vi "FipsAdjacent.vi"() -> (11 "Fips":i32[](array[numeric]))   [LabVIEW 2017] (continued)
 County, TX\"\t48317\n\"Glasscock County, TX\"\t48173\t\"Midland County, TX\"\t48329\n\"Glasscock County, TX\"\t48173\t\"Reagan County, TX\"\t48383\n\"Glasscock County, TX\"\t48173\t\"Sterling County, TX\"\t48431\n\"Glasscock County, TX\"\t48173\t\"Upton County, TX\"\t48461\n\"Goliad County, TX\"\t48175\t\"Bee County, TX\"\t48025\n\"Goliad County, TX\"\t48175\t\"DeWitt County, TX\"\t48123\n\"Goliad County, TX\"\t48175\t\"Goliad County, TX\"\t48175\n\"Goliad County, TX\"\t48175\t\"Karnes County, TX\"\t48255\n\"Goliad County, TX\"\t48175\t\"Refugio County, TX\"\t48391\n\"Goliad County, TX\"\t48175\t\"Victoria County, TX\"\t48469\n\"Gonzales County, TX\"\t48177\t\"Caldwell County, TX\"\t48055\n\"Gonzales County, TX\"\t48177\t\"DeWitt County, TX\"\t48123\n\"Gonzales County, TX\"\t48177\t\"Fayette County, TX\"\t48149\n\"Gonzales County, TX\"\t48177\t\"Gonzales County, TX\"\t48177\n\"Gonzales County, TX\"\t48177\t\"Guadalupe County, TX\"\t48187\n\"Gonzales County, TX\"\t48177\t\"Karnes County, TX\"\t48255\n\"Gonzales County, TX\"\t48177\t\"Lavaca County, TX\"\t48285\n\"Gonzales County, TX\"\t48177\t\"Wilson County, TX\"\t48493\n\"Gray County, TX\"\t48179\t\"Armstrong County, TX\"\t48011\n\"Gray County, TX\"\t48179\t\"Carson County, TX\"\t48065\n\"Gray County, TX\"\t48179\t\"Collingsworth County, TX\"\t48087\n\"Gray County, TX\"\t48179\t\"Donley County, TX\"\t48129\n\"Gray County, TX\"\t48179\t\"Gray County, TX\"\t48179\n\"Gray County, TX\"\t48179\t\"Hemphill County, TX\"\t48211\n\"Gray County, TX\"\t48179\t\"Roberts County, TX\"\t48393\n\"Gray County, TX\"\t48179\t\"Wheeler County, TX\"\t48483\n\"Grayson County, TX\"\t48181\t\"Bryan County, OK\"\t40013\n\"Grayson County, TX\"\t48181\t\"Love County, OK\"\t40085\n\"Grayson County, TX\"\t48181\t\"Marshall County, OK\"\t40095\n\"Grayson County, TX\"\t48181\t\"Collin County, TX\"\t48085\n\"Grayson County, TX\"\t48181\t\"Cooke County, TX\"\t48097\n\"Grayson County, TX\"\t48181\t\"Denton County, TX\"\t48121\n\"Grayson County, TX\"\t48181\t\"Fannin County, TX\"\t48147\n\"Grayson County, TX\"\t48181\t\"Grayson County, TX\"\t48181\n\"Gregg County, TX\"\t48183\t\"Gregg County, TX\"\t48183\n\"Gregg County, TX\"\t48183\t\"Harrison County, TX\"\t48203\n\"Gregg County, TX\"\t48183\t\"Rusk County, TX\"\t48401\n\"Gregg County, TX\"\t48183\t\"Smith County, TX\"\t48423\n\"Gregg County, TX\"\t48183\t\"Upshur County, TX\"\t48459\n\"Grimes County, TX\"\t48185\t\"Brazos County, TX\"\t48041\n\"Grimes County, TX\"\t48185\t\"Grimes County, TX\"\t48185\n\"Grimes County, TX\"\t48185\t\"Madison County, TX\"\t48313\n\"Grimes County, TX\"\t48185\t\"Montgomery County, TX\"\t48339\n\"Grimes County, TX\"\t48185\t\"Walker County, TX\"\t48471\n\"Grimes County, TX\"\t48185\t\"Waller County, TX\"\t48473\n\"Grimes County, TX\"\t48185\t\"Washington County, TX\"\t48477\n\"Guadalupe County, TX\"\t48187\t\"Bexar County, TX\"\t48029\n\"Guadalupe County, TX\"\t48187\t\"Caldwell County, TX\"\t48055\n\"Guadalupe County, TX\"\t48187\t\"Comal County, TX\"\t48091\n\"Guadalupe County, TX\"\t48187\t\"Gonzales County, TX\"\t48177\n\"Guadalupe County, TX\"\t48187\t\"Guadalupe County, TX\"\t48187\n\"Guadalupe County, TX\"\t48187\t\"Hays County, TX\"\t48209\n\"Guadalupe County, TX\"\t48187\t\"Wilson County, TX\"\t48493\n\"Hale County, TX\"\t48189\t\"Castro County, TX\"\t48069\n\"Hale County, TX\"\t48189\t\"Crosby County, TX\"\t48107\n\"Hale County, TX\"\t48189\t\"Floyd County, TX\"\t48153\n\"Hale County, TX\"\t48189\t\"Hale County, TX\"\t48189\n\"Hale County, TX\"\t48189\t\"Hockley County, TX\"\t48219\n\"Hale County, TX\"\t48189\t\"Lamb County, TX\"\t48279\n\"Hale County, TX\"\t48189\t\"Lubbock County, TX\"\t48303\n\"Hale County, TX\"\t48189\t\"Swisher County, TX\"\t48437\n\"Hall County, TX\"\t48191\t\"Briscoe County, TX\"\t48045\n\"Hall County, TX\"\t48191\t\"Childress County, TX\"\t48075\n\"Hall County, TX\"\t48191\t\"Collingsworth County, TX\"\t48087\n\"Hall County, TX\"\t48191\t\"Cottle County, TX\"\t48101\n\"Hall County, TX\"\t48191\t\"Donley County, TX\"\t48129\n\"Hall County, TX\"\t48191\t\"Hall County, TX\"\t48191\n\"Hall County, TX\"\t48191\t\"Motley County, TX\"\t48345\n\"Hamilton County, TX\"\t48193\t\"Bosque County, TX\"\t48035\n\"Hamilton County, TX\"\t48193\t\"Comanche County, TX\"\t48093\n\"Hamilton County, TX\"\t48193\t\"Coryell County, TX\"\t48099\n\"Hamilton County, TX\"\t48193\t\"Erath County, TX\"\t48143\n\"Hamilton County, TX\"\t48193\t\"Hamilton County, TX\"\t48193\n\"Hamilton County, TX\"\t48193\t\"Lampasas County, TX\"\t48281\n\"Hamilton County, TX\"\t48193\t\"Mills County, TX\"\t48333\n\"Hansford County, TX\"\t48195\t\"Texas County, OK\"\t40139\n\"Hansford County, TX\"\t48195\t\"Hansford County, TX\"\t48195\n\"Hansford County, TX\"\t48195\t\"Hutchinson County, TX\"\t48233\n\"Hansford County, TX\"\t48195\t\"Moore County, TX\"\t48341\n\"Hansford County, TX\"\t48195\t\"Ochiltree County, TX\"\t48357\n\"Hansford County, TX\"\t48195\t\"Roberts County, TX\"\t48393\n\"Hansford County, TX\"\t48195\t\"Sherman County, TX\"\t48421\n\"Hardeman County, TX\"\t48197\t\"Harmon County, OK\"\t40057\n\"Hardeman County, TX\"\t48197\t\"Jackson County, OK\"\t40065\n\"Hardeman County, TX\"\t48197\t\"Childress County, TX\"\t48075\n\"Hardeman County, TX\"\t48197\t\"Cottle County, TX\"\t48101\n\"Hardeman County, TX\"\t48197\t\"Foard County, TX\"\t48155\n\"Hardeman County, TX\"\t48197\t\"Hardeman County, TX\"\t48197\n\"Hardeman County, TX\"\t48197\t\"Wilbarger County, TX\"\t48487\n\"Hardin County, TX\"\t48199\t\"Hardin County, TX\"\t48199\n\"Hardin County, TX\"\t48199\t\"Jasper County, TX\"\t48241\n\"Hardin County, TX\"\t48199\t\"Jefferson County, TX\"\t48245\n\"Hardin County, TX\"\t48199\t\"Liberty County, TX\"\t48291\n\"Hardin County, TX\"\t48199\t\"Orange County, TX\"\t48361\n\"Hardin County, TX\"\t48199\t\"Polk County, TX\"\t48373\n\"Hardin County, TX\"\t48199\t\"Tyler County, TX\"\t48457\n\"Harris County, TX\"\t48201\t\"Brazoria County, TX\"\t48039\n\"Harris County, TX\"\t48201\t\"Chambers County, TX\"\t48071\n\"Harris County, TX\"\t48201\t\"Fort Bend County, TX\"\t48157\n\"Harris County, TX\"\t48201\t\"Galveston County, TX\"\t48167\n\"Harris County, TX\"\t48201\t\"Harris County, TX\"\t48201\n\"Harris County, TX\"\t48201\t\"Liberty County, TX\"\t48291\n\"Harris County, TX\"\t48201\t\"Montgomery County, TX\"\t48339\n\"Harris County, TX\"\t48201\t\"Waller County, TX\"\t48473\n\"Harrison County, TX\"\t48203\t\"Caddo Parish, LA\"\t22017\n\"Harrison County, TX\"\t48203\t\"Gregg County, TX\"\t48183\n\"Harrison County, TX\"\t48203\t\"Harrison County, TX\"\t48203\n\"Harrison County, TX\"\t48203\t\"Marion County, TX\"\t48315\n\"Harrison County, TX\"\t48203\t\"Panola County, TX\"\t48365\n\"Harrison County, TX\"\t48203\t\"Rusk County, TX\"\t48401\n\"Harrison County, TX\"\t48203\t\"Upshur County, TX\"\t48459\n\"Hartley County, TX\"\t48205\t\"Quay County, NM\"\t35037\n\"Hartley County, TX\"\t48205\t\"Union County, NM\"\t35059\n\"Hartley County, TX\"\t48205\t\"Dallam County, TX\"\t48111\n\"Hartley County, TX\"\t48205\t\"Hartley County, TX\"\t48205\n\"Hartley County, TX\"\t48205\t\"Moore County, TX\"\t48341\n\"Hartley County, TX\"\t48205\t\"Oldham County, TX\"\t48359\n\"Hartley County, TX\"\t48205\t\"Sherman County, TX\"\t48421\n\"Haskell County, TX\"\t48207\t\"Baylor County, TX\"\t48023\n\"Haskell County, TX\"\t48207\t\"Haskell County, TX\"\t48207\n\"Haskell County, TX\"\t48207\t\"Jones County, TX\"\t48253\n\"Haskell County, TX\"\t48207\t\"King County, TX\"\t48269\n\"Haskell County, TX\"\t48207\t\"Knox County, TX\"\t48275\n\"Haskell County, TX\"\t48207\t\"Shackelford County, TX\"\t48417\n\"Haskell County, TX\"\t48207\t\"Stonewall County, TX\"\t48433\n\"Haskell County, TX\"\t48207\t\"Throckmorton County, TX\"\t48447\n\"Hays County, TX\"\t48209\t\"Blanco County, TX\"\t48031\n\"Hays County, TX\"\t48209\t\"Caldwell County, TX\"\t48055\n\"Hays County, TX\"\t48209\t\"Comal County, TX\"\t48091\n\"Hays County, TX\"\t48209\t\"Guadalupe County, TX\"\t48187\n\"Hays County, TX\"\t48209\t\"Hays County, TX\"\t48209\n\"Hays County, TX\"\t48209\t\"Travis County, TX\"\t48453\n\"Hemphill County, TX\"\t48211\t\"Ellis County, OK\"\t40045\n\"Hemphill County, TX\"\t48211\t\"Roger Mills County, OK\"\t40129\n\"Hemphill County, TX\"\t48211\t\"Gray County, TX\"\t48179\n\"Hemphill County, TX\"\t48211\t\"Hemphill County, TX\"\t48211\n\"Hemphill County, TX\"\t48211\t\"Lipscomb County, TX\"\t48295\n\"Hemphill County, TX\"\t48211\t\"Roberts County, TX\"\t48393\n\"Hemphill County, TX\"\t48211\t\"Wheeler County, TX\"\t48483\n\"Henderson County, TX\"\t48213\t\"Anderson County, TX\"\t48001\n\"Henderson County, TX\"\t48213\t\"Cherokee County, TX\"\t48073\n\"Henderson County, TX\"\t48213\t\"Ellis County, TX\"\t48139\n\"Henderson County, TX\"\t48213\t\"Freestone County, TX\"\t48161\n\"Henderson County, TX\"\t48213\t\"Henderson County, TX\"\t48213\n\"Henderson County, TX\"\t48213\t\"Kaufman County, TX\"\t48257\n\"Henderson County, TX\"\t48213\t\"Navarro County, TX\"\t48349\n\"Henderson County, TX\"\t48213\t\"Smith County, TX\"\t48423\n\"Henderson County, TX\"\t48213\t\"Van Zandt County, TX\"\t48467\n\"Hidalgo County, TX\"\t48215\t\"Brooks County, TX\"\t48047\n\"Hidalgo County, TX\"\t48215\t\"Cameron County, TX\"\t48061\n\"Hidalgo County, TX\"\t48215\t\"Hidalgo County, TX\"\t48215\n\"Hidalgo County, TX\"\t48215\t\"Kenedy County, TX\"\t48261\n\"Hidalgo County, TX\"\t48215\t\"Starr County, TX\"\t48427\n\"Hidalgo County, TX\"\t48215\t\"Willacy County, TX\"\t48489\n\"Hill County, TX\"\t48217\t\"Bosque County, TX\"\t48035\n\"Hill County, TX\"\t48217\t\"Ellis County, TX\"\t48139\n\"Hill County, TX\"\t48217\t\"Hill County, TX\"\t48217\n\"Hill County, TX\"\t48217\t\"Johnson County, TX\"\t48251\n\"Hill County, TX\"\t48217\t\"Limestone County, TX\"\t48293\n\"Hill County, TX\"\t48217\t\"McLennan County, TX\"\t48309\n\"Hill County, TX\"\t48217\t\"Navarro County, TX\"\t48349\n\"Hockley County, TX\"\t48219\t\"Bailey County, TX\"\t48017\n\"Hockley County, TX\"\t48219\t\"Cochran County, TX\"\t48079\n\"Hockley County, TX\"\t48219\t\"Hale County, TX\"\t48189\n\"Hockley County, TX\"\t48219\t\"Hockley County, TX\"\t48219\n\"Hockley County, TX\"\t48219\t\"Lamb County, TX\"\t48279\n\"Hockley County, TX\"\t48219\t\"Lubbock County, TX\"\t48303\n\"Hockley County, TX\"\t48219\t\"Lynn County, TX\"\t48305\n\"Hockley County, TX\"\t48219\t\"Terry County, TX\"\t48445\n\"Hockley County, TX\"\t48219\t\"Yoakum County, TX\"\t48501\n\"Hood County, TX\"\t48221\t\"Erath County, TX\"\t48143\n\"Hood County, TX\"\t48221\t\"Hood County, TX\"\t48221\n\"Hood County, TX\"\t48221\t\"Johnson County, TX\"\t48251\n\"Hood County, TX\"\t48221\t\"Palo Pinto County, TX\"\t48363\n\"Hood County, TX\"\t48221\t\"Parker County, TX\"\t48367\n\"Hood County, TX\"\t48221\t\"Somervell County, TX\"\t48425\n\"Hopkins County, TX\"\t48223\t\"Delta County, TX\"\t48119\n\"Hopkins County, TX\"\t48223\t\"Franklin County, TX\"\t48159\n\"Hopkins County, TX\"\t48223\t\"Hopkins County, TX\"\t48223\n\"Hopkins County, TX\"\t48223\t\"Hunt County, TX\"\t48231\n\"Hopkins County, TX\"\t48223\t\"Rains County, TX\"\t48379\n\"Hopkins County, TX\"\t48223\t\"Wood County, TX\"\t48499\n\"Houston County, TX\"\t48225\t\"Anderson County, TX\"\t48001\n\"Houston County, TX\"\t48225\t\"Angelina County, TX\"\t48005\n\"Houston County, TX\"\t48225\t\"Cherokee County, TX\"\t48073\n\"Houston County, TX\"\t48225\t\"Houston County, TX\"\t48225\n\"Houston County, TX\"\t48225\t\"Leon County, TX\"\t48289\n\"Houston County, TX\"\t48225\t\"Madison County, TX\"\t48313\n\"Houston County, TX\"\t48225\t\"Trinity County, TX\"\t48455\n\"Houston County, TX\"\t48225\t\"Walker County, TX\"\t48471\n\"Howard County, TX\"\t48227\t\"Borden County, TX\"\t48033\n\"Howard County, TX\"\t48227\t\"Dawson County, TX\"\t48115\n\"Howard County, TX\"\t48227\t\"Glasscock County, TX\"\t48173\n\"Howard County, TX\"\t48227\t\"Howard County, TX\"\t48227\n\"Howard County, TX\"\t48227\t\"Martin County, TX\"\t48317\n\"Howard County, TX\"\t48227\t\"Mitchell County, TX\"\t48335\n\"Howard County, TX\"\t48227\t\"Sterling County, TX\"\t48431\n\"Hudspeth County, TX\"\t48229\t\"Otero County, NM\"\t35035\n\"Hudspeth County, TX\"\t48229\t\"Culberson County, TX\"\t48109\n\"Hudspeth County, TX\"\t48229\t\"El Paso County, TX\"\t48141\n\"Hudspeth County, TX\"\t48229\t\"Hudspeth County, TX\"\t48229\n\"Hudspeth County, TX\"\t48229\t\"Jeff Davis County, TX\"\t48243\n\"Hudspeth County, TX\"\t48229\t\"Presidio County, TX\"\t48377\n\"Hunt County, TX\"\t48231\t\"Collin County, TX\"\t48085\n\"Hunt County, TX\"\t48231\t\"Delta County, TX\"\t48119\n\"Hunt County, TX\"\t48231\t\"Fannin County, TX\"\t48147\n\"Hunt County, TX\"\t48231\t\"Hopkins County, TX\"\t48223\n\"Hunt County, TX\"\t48231\t\"Hunt County, TX\"\t48231\n\"Hunt County, TX\"\t48231\t\"Kaufman County, TX\"\t48257\n\"Hunt County, TX\"\t48231\t\"Rains County, TX\"\t48379\n\"Hunt County, TX\"\t48231\t\"Rockwall County, TX\"\t48397\n\"Hunt County, TX\"\t48231\t\"Van Zandt County, TX\"\t48467\n\"Hutchinson County, TX\"\t48233\t\"Carson County, TX\"\t48065\n\"Hutchinson County, TX\"\t48233\t\"Hansford County, TX\"\t48195\n\"Hutchinson County, TX\"\t48233\t\"Hutchinson County, TX\"\t48233\n\"Hutchinson County, TX\"\t48233\t\"Moore County, TX\"\t48341\n\"Hutchinson County, TX\"\t48233\t\"Roberts County, TX\"\t48393\n\"Hutchinson County, TX\"\t48233\t\"Sherman County, TX\"\t48421\n\"Irion County, TX\"\t48235\t\"Crockett County, TX\"\t48105\n\"Irion County, TX\"\t48235\t\"Irion County, TX\"\t48235\n\"Irion County, TX\"\t48235\t\"Reagan County, TX\"\t48383\n\"Irion County, TX\"\t48235\t\"Schleicher County, TX\"\t48413\n\"Irion County, TX\"\t48235\t\"Tom Green County, TX\"\t48451\n\"Jack County, TX\"\t48237\t\"Archer County, TX\"\t48009\n\"Jack County, TX\"\t48237\t\"Clay County, TX\"\t48077\n\"Jack County, TX\"\t48237\t\"Jack County, TX\"\t48237\n\"Jack County, TX\"\t48237\t\"Montague County, TX\"\t48337\n\"Jack County, TX\"\t48237\t\"Palo Pinto County, TX\"\t48363\n\"Jack County, TX\"\t48237\t\"Parker County, TX\"\t48367\n\"Jack County, TX\"\t48237\t\"Wise County, TX\"\t48497\n\"Jack County, TX\"\t48237\t\"Young County, TX\"\t48503\n\"Jackson County, TX\"\t48239\t\"Calhoun County, TX\"\t48057\n\"Jackson County, TX\"\t48239\t\"Colorado County, TX\"\t48089\n\"Jackson County, TX\"\t48239\t\"Jackson County, TX\"\t48239\n\"Jackson County, TX\"\t48239\t\"Lavaca County, TX\"\t48285\n\"Jackson County, TX\"\t48239\t\"Matagorda County, TX\"\t48321\n\"Jackson County, TX\"\t48239\t\"Victoria County, TX\"\t48469\n\"Jackson County, TX\"\t48239\t\"Wharton County, TX\"\t48481\n\"Jasper County, TX\"\t48241\t\"Angelina County, TX\"\t48005\n\"Jasper County, TX\"\t48241\t\"Hardin County, TX\"\t48199\n\"Jasper County, TX\"\t48241\t\"Jasper County, TX\"\t48241\n\"Jasper County, TX\"\t48241\t\"Newton County, TX\"\t48351\n\"Jasper County, TX\"\t48241\t\"Orange County, TX\"\t48361\n\"Jasper County, TX\"\t48241\t\"Sabine County, TX\"\t48403\n\"Jasper County, TX\"\t48241\t\"San Augustine County, TX\"\t48405\n\"Jasper County, TX\"\t48241\t\"Tyler County, TX\"\t48457\n\"Jeff Davis County, TX\"\t48243\t\"Brewster County, TX\"\t48043\n\"Jeff Davis County, TX\"\t48243\t\"Culberson County, TX\"\t48109\n\"Jeff Davis County, TX\"\t48243\t\"Hudspeth County, TX\"\t48229\n\"Jeff Davis County, TX\"\t48243\t\"Jeff Davis County, TX\"\t48243\n\"Jeff Davis County, TX\"\t48243\t\"Pecos County, TX\"\t48371\n\"Jeff Davis County, TX\"\t48243\t\"Presidio County, TX\"\t48377\n\"Jeff Davis County, TX\"\t48243\t\"Reeves County, TX\"\t48389\n\"Jefferson County, TX\"\t48245\t\"Cameron Parish, LA\"\t22023\n\"Jefferson County, TX\"\t48245\t\"Chambers County, TX\"\t48071\n\"Jefferson County, TX\"\t48245\t\"Hardin County, TX\"\t48199\n\"Jefferson County, TX\"\t48245\t\"Jefferson County, TX\"\t48245\n\"Jefferson County, TX\"\t48245\t\"Liberty County, TX\"\t48291\n\"Jefferson County, TX\"\t48245\t\"Orange County, TX\"\t48361\n\"Jim Hogg County, TX\"\t48247\t\"Brooks County, TX\"\t48047\n\"Jim Hogg County, TX\"\t48247\t\"Duval County, TX\"\t48131\n\"Jim Hogg County, TX\"\t48247\t\"Jim Hogg County, TX\"\t48247\n\"Jim Hogg County, TX\"\t48247\t\"Starr County, TX\"\t48427\n\"Jim Hogg County, TX\"\t48247\t\"Webb County, TX\"\t48479\n\"Jim Hogg County, TX\"\t48247\t\"Zapata County, TX\"\t48505\n\"Jim Wells County, TX\"\t48249\t\"Brooks County, TX\"\t48047\n\"Jim Wells County, TX\"\t48249\t\"Duval County, TX\"\t48131\n\"Jim Wells County, TX\"\t48249\t\"Jim Wells County, TX\"\t48249\n\"Jim Wells County, TX\"\t48249\t\"Kleberg County, TX\"\t48273\n\"Jim Wells County, TX\"\t48249\t\"Live Oak County, TX\"\t48297\n\"Jim Wells County, TX\"\t48249\t\"Nueces County, TX\"\t48355\n\"Jim Wells County, TX\"\t48249\t\"San Patricio County, TX\"\t48409\n\"Johnson County, TX\"\t48251\t\"Bosque County, TX\"\t48035\n\"Johnson County, TX\"\t48251\t\"Ellis County, TX\"\t48139\n\"Johnson County, TX\"\t48251\t\"Hill County, TX\"\t48217\n\"Johnson County, TX\"\t48251\t\"Hood County, TX\"\t48221\n\"Johnson County, TX\"\t48251\t\"Johnson County, TX\"\t48251\n\"Johnson County, TX\"\t48251\t\"Parker County, TX\"\t48367\n\"Johnson County, TX\"\t48251\t\"Somervell County, TX\"\t48425\n\"Johnson County, TX\"\t48251\t\"Tarrant County, TX\"\t48439\n\"Jones County, TX\"\t48253\t\"Callahan County, TX\"\t48059\n\"Jones County, TX\"\t48253\t\"Fisher County, TX\"\t48151\n\"Jones County, TX\"\t48253\t\"Haskell County, TX\"\t48207\n\"Jones County, TX\"\t48253\t\"Jones County, TX\"\t48253\n\"Jones County, TX\"\t48253\t\"Nolan County, TX\"\t48353\n\"Jones County, TX\"\t48253\t\"Shackelford County, TX\"\t48417\n\"Jones County, TX\"\t48253\t\"Stonewall County, TX\"\t48433\n\"Jones County, TX\"\t48253\t\"Taylor County, TX\"\t48441\n\"Karnes County, TX\"\t48255\t\"Atascosa County, TX\"\t48013\n\"Karnes County, TX\"\t48255\t\"Bee County, TX\"\t48025\n\"Karnes County, TX\"\t48255\t\"DeWitt County, TX\"\t48123\n\"Karnes County, TX\"\t48255\t\"Goliad County, TX\"\t48175\n\"Karnes County, TX\"\t48255\t\"Gonzales County, TX\"\t48177\n\"Karnes County, TX\"\t48255\t\"Karnes County, TX\"\t48255\n\"Karnes County, TX\"\t48255\t\"Live Oak County, TX\"\t48297\n\"Karnes County, TX\"\t48255\t\"Wilson County, TX\"\t48493\n\"Kaufman County, TX\"\t48257\t\"Dallas County, TX\"\t48113\n\"Kaufman County, TX\"\t48257\t\"Ellis County, TX\"\t48139\n\"Kaufman County, TX\"\t48257\t\"Henderson County, TX\"\t48213\n\"Kaufman County, TX\"\t48257\t\"Hunt County, TX\"\t48231\n\"Kaufman County, TX\"\t48257\t\"Kaufman County, TX\"\t48257\n\"Kaufman County, TX\"\t48257\t\"Rockwall County, TX\"\t48397\n\"Kaufman County, TX\"\t48257\t\"Van Zandt County, TX\"\t48467\n\"Kendall County, TX\"\t48259\t\"Bandera County, TX\"\t48019\n\"Kendall County, TX\"\t48259\t\"Bexar County, TX\"\t48029\n\"Kendall County, TX\"\t48259\t\"Blanco County, TX\"\t48031\n\"Kendall County, TX\"\t48259\t\"Comal County, TX\"\t48091\n\"Kendall County, TX\"\t48259\t\"Gillespie County, TX\"\t48171\n\"Kendall County, TX\"\t48259\t\"Kendall County, TX\"\t48259\n\"Kendall County, TX\"\t48259\t\"Kerr County, TX\"\t48265\n\"Kenedy County, TX\"\t48261\t\"Brooks County, TX\"\t48047\n\"Kenedy County, TX\"\t48261\t\"Hidalgo County, TX\"\t48215\n\"Kenedy County, TX\"\t48261\t\"Kenedy County, TX\"\t48261\n\"Kenedy County, TX\"\t48261\t\"Kleberg County, TX\"\t48273\n\"Kenedy County, TX\"\t48261\t\"Willacy County, TX\"\t48489\n\"Kent County, TX\"\t48263\t\"Crosby County, TX\"\t48107\n\"Kent County, TX\"\t48263\t\"Dickens County, TX\"\t48125\n\"Kent County, TX\"\t48263\t\"Fisher County, TX\"\t48151\n\"Kent County, TX\"\t48263\t\"Garza County, TX\"\t48169\n\"Kent County, TX\"\t48263\t\"Kent County, TX\"\t48263\n\"Kent County, TX\"\t48263\t\"King County, TX\"\t48269\n\"Kent County, TX\"\t48263\t\"Scurry County, TX\"\t48415\n\"Kent County, TX\"\t48263\t\"Stonewall County, TX\"\t48433\n\"Kerr County, TX\"\t48265\t\"Bandera County, TX\"\t48019\n\"Kerr County, TX\"\t48265\t\"Edwards County, TX\"\t48137\n\"Kerr County, TX\"\t48265\t\"Gillespie County, TX\"\t48171\n\"Kerr County, TX\"\t48265\t\"Kendall County, TX\"\t48259\n\"Kerr County, TX\"\t48265\t\"Kerr County, TX\"\t48265\n\"Kerr County, TX\"\t48265\t\"Kimble County, TX\"\t48267\n\"Kerr County, TX\"\t48265\t\"Real County, TX\"\t48385\n\"Kimble County, TX\"\t48267\t\"Edwards County, TX\"\t48137\n\"Kimble County, TX\"\t48267\t\"Gillespie County, TX\"\t48171\n\"Kimble County, TX\"\t48267\t\"Kerr County, TX\"\t48265\n\"Kimble County, TX\"\t48267\t\"Kimble County, TX\"\t48267\n\"Kimble County, TX\"\t48267\t\"Mason County, TX\"\t48319\n\"Kimble County, TX\"\t48267\t\"Menard County, TX\"\t48327\n\"Kimble County, TX\"\t48267\t\"Schleicher County, TX\"\t48413\n\"Kimble County, TX\"\t48267\t\"Sutton County, TX\"\t48435\n\"King County, TX\"\t48269\t\"Cottle County, TX\"\t48101\n\"King County, TX\"\t48269\t\"Dickens County, TX\"\t48125\n\"King County, TX\"\t48269\t\"Foard County, TX\"\t48155\n\"King County, TX\"\t48269\t\"Haskell County, TX\"\t48207\n\"King County, TX\"\t48269\t\"Kent County, TX\"\t48263\n\"King County, TX\"\t48269\t\"King County, TX\"\t48269\n\"King County, TX\"\t48269\t\"Knox County, TX\"\t48275\n\"King County, TX\"\t48269\t\"Motley County, TX\"\t48345\n\"King County, TX\"\t48269\t\"Stonewall County, TX\"\t48433\n\"Kinney County, TX\"\t48271\t\"Edwards County, TX\"\t48137\n\"Kinney County, TX\"\t48271\t\"Kinney County, TX\"\t48271\n\"Kinney County, TX\"\t48271\t\"Maverick County, TX\"\t48323\n\"Kinney County, TX\"\t48271\t\"Uvalde County, TX\"\t48463\n\"Kinney County, TX\"\t48271\t\"Val Verde County, TX\"\t48465\n\"Kinney County, TX\"\t48271\t\"Zavala County, TX\"\t48507\n\"Kleberg County, TX\"\t48273\t\"Brooks County, TX\"\t48047\n\"Kleberg County, TX\"\t48273\t\"Jim Wells County, TX\"\t48249\n\"Kleberg County, TX\"\t48273\t\"Kenedy County, TX\"\t48261\n\"Kleberg County, TX\"\t48273\t\"Kleberg County, TX\"\t48273\n\"Kleberg County, TX\"\t48273\t\"Nueces County, TX\"\t48355\n\"Knox County, TX\"\t48275\t\"Baylor County, TX\"\t48023\n\"Knox County, TX\"\t48275\t\"Foard County, TX\"\t48155\n\"Knox County, TX\"\t48275\t\"Haskell County, TX\"\t48207\n\"Knox County, TX\"\t48275\t\"King County, TX\"\t48269\n\"Knox County, TX\"\t48275\t\"Knox County, TX\"\t48275\n\"Knox County, TX\"\t48275\t\"Stonewall County, TX\"\t48433\n\"Knox County, TX\"\t48275\t\"Throckmorton County, TX\"\t48447\n\"Lamar County, TX\"\t48277\t\"Bryan County, OK\"\t40013\n\"Lamar County, TX\"\t48277\t\"Choctaw County, OK\"\t40023\n\"Lamar County, TX\"\t48277\t\"Delta County, TX\"\t48119\n\"Lamar County, TX\"\t48277\t\"Fannin County, TX\"\t48147\n\"Lamar County, TX\"\t48277\t\"Lamar County, TX\"\t48277\n\"Lamar County, TX\"\t48277\t\"Red River County, TX\"\t48387\n\"Lamb County, TX\"\t48279\t\"Bailey County, TX\"\t48017\n\"Lamb County, TX\"\t48279\t\"Castro County, TX\"\t48069\n\"Lamb County, TX\"\t48279\t\"Cochran County, TX\"\t48079\n\"Lamb County, TX\"\t48279\t\"Hale County, TX\"\t48189\n\"Lamb County, TX\"\t48279\t\"Hockley County, TX\"\t48219\n\"Lamb County, TX\"\t48279\t\"Lamb County, TX\"\t48279\n\"Lamb County, TX\"\t48279\t\"Lubbock County, TX\"\t48303\n\"Lamb County, TX\"\t48279\t\"Parmer County, TX\"\t48369\n\"Lampasas County, TX\"\t48281\t\"Bell County, TX\"\t48027\n\"Lampasas County, TX\"\t48281\t\"Burnet County, TX\"\t48053\n\"Lampasas County, TX\"\t48281\t\"Coryell County, TX\"\t48099\n\"Lampasas County, TX\"\t48281\t\"Hamilton County, TX\"\t48193\n\"Lampasas County, TX\"\t48281\t\"Lampasas County, TX\"\t48281\n\"Lampasas County, TX\"\t48281\t\"Mills County, TX\"\t48333\n\"Lampasas County, TX\"\t48281\t\"San Saba County, TX\"\t48411\n\"La Salle County, TX\"\t48283\t\"Atascosa County, TX\"\t48013\n\"La Salle County, TX\"\t48283\t\"Dimmit County, TX\"\t48127\n\"La Salle County, TX\"\t48283\t\"Duval County, TX\"\t48131\n\"La Salle County, TX\"\t48283\t\"Frio County, TX\"\t48163\n\"La Salle County, TX\"\t48283\t\"La Salle County, TX\"\t48283\n\"La Salle County, TX\"\t48283\t\"McMullen County, TX\"\t48311\n\"La Salle County, TX\"\t48283\t\"Webb County, TX\"\t48479\n\"Lavaca County, TX\"\t48285\t\"Colorado County, TX\"\t48089\n\"Lavaca County, TX\"\t48285\t\"DeWitt County, TX\"\t48123\n\"Lavaca County, TX\"\t48285\t\"Fayette County, TX\"\t48149\n\"Lavaca County, TX\"\t48285\t\"Gonzales County, TX\"\t48177\n\"Lavaca County, TX\"\t48285\t\"Jackson County, TX\"\t48239\n\"Lavaca County, TX\"\t48285\t\"Lavaca County, TX\"\t48285\n\"Lavaca County, TX\"\t48285\t\"Victoria County, TX\"\t48469\n\"Lee County, TX\"\t48287\t\"Bastrop County, TX\"\t48021\n\"Lee County, TX\"\t48287\t\"Burleson County, TX\"\t48051\n\"Lee County, TX\"\t48287\t\"Fayette County, TX\"\t48149\n\"Lee County, TX\"\t48287\t\"Lee County, TX\"\t48287\n\"Lee County, TX\"\t48287\t\"Milam County, TX\"\t48331\n\"Lee County, TX\"\t48287\t\"Washington County, TX\"\t48477\n\"Lee County, TX\"\t48287\t\"Williamson County, TX\"\t48491\n\"Leon County, TX\"\t48289\t\"Anderson County, TX\"\t48001\n\"Leon County, TX\"\t48289\t\"Brazos County, TX\"\t48041\n\"Leon County, TX\"\t48289\t\"Freestone County, TX\"\t48161\n\"Leon County, TX\"\t48289\t\"Houston County, TX\"\t48225\n\"Leon County, TX\"\t48289\t\"Leon County, TX\"\t48289\n\"Leon County, TX\"\t48289\t\"Limestone County, TX\"\t48293\n\"Leon County, TX\"\t48289\t\"Madison County, TX\"\t48313\n\"Leon County, TX\"\t48289\t\"Robertson County, TX\"\t48395\n\"Liberty County, TX\"\t48291\t\"Chambers County, TX\"\t48071\n\"Liberty County, TX\"\t48291\t\"Hardin County, TX\"\t48199\n\"Liberty County, TX\"\t48291\t\"Harris County, TX\"\t48201\n\"Liberty County, TX\"\t48291\t\"Jefferson County, TX\"\t48245\n\"Liberty County, TX\"\t48291\t\"Liberty County, TX\"\t48291\n\"Liberty County, TX\"\t48291\t\"Montgomery County, TX\"\t48339\n\"Liberty County, TX\"\t48291\t\"Polk County, TX\"\t48373\n\"Liberty County, TX\"\t48291\t\"San Jacinto County, TX\"\t48407\n\"Limestone County, TX\"\t48293\t\"Falls County, TX\"\t48145\n\"Limestone County, TX\"\t48293\t\"Freestone County, TX\"\t48161\n\"Limestone County, TX\"\t48293\t\"Hill County, TX\"\t48217\n\"Limestone County, TX\"\t48293\t\"Leon County, TX\"\t48289\n\"Limestone County, TX\"\t48293\t\"Limestone County, TX\"\t48293\n\"Limestone County, TX\"\t48293\t\"McLennan County, TX\"\t48309\n\"Limestone County, TX\"\t48293\t\"Navarro County, TX\"\t48349\n\"Limestone County, TX\"\t48293\t\"Robertson County, TX\"\t48395\n\"Lipscomb County, TX\"\t48295\t\"Beaver County, OK\"\t40007\n\"Lipscomb County, TX\"\t48295\t\"Ellis County, OK\"\t40045\n\"Lipscomb County, TX\"\t48295\t\"Hemphill County, TX\"\t48211\n\"Lipscomb County, TX\"\t48295\t\"Lipscomb County, TX\"\t48295\n\"Lipscomb County, TX\"\t48295\t\"Ochiltree County, TX\"\t48357\n\"Lipscomb County, TX\"\t48295\t\"Roberts County, TX\"\t48393\n\"Live Oak County, TX\"\t48297\t\"Atascosa County, TX\"\t48013\n\"Live Oak County, TX\"\t48297\t\"Bee County, TX\"\t48025\n\"Live Oak County, TX\"\t48297\t\"Duval County, TX\"\t48131\n\"Live Oak County, TX\"\t48297\t\"Jim Wells County, TX\"\t48249\n\"Live Oak County, TX\"\t48297\t\"Karnes County, TX\"\t48255\n\"Live Oak County, TX\"\t48297\t\"Live Oak County, TX\"\t48297\n\"Live Oak County, TX\"\t48297\t\"McMullen County, TX\"\t48311\n\"Live Oak County, TX\"\t48297\t\"San Patricio County, TX\"\t48409\n\"Llano County, TX\"\t48299\t\"Blanco County, TX\"\t48031\n\"Llano County, TX\"\t48299\t\"Burnet County, TX\"\t48053\n\"Llano County, TX\"\t48299\t\"Gillespie County, TX\"\t48171\n\"Llano County, TX\"\t48299\t\"Llano County, TX\"\t48299\n\"Llano County, TX\"\t48299\t\"Mason County, TX\"\t48319\n\"Llano County, TX\"\t48299\t\"San Saba County, TX\"\t48411\n\"Loving County, TX\"\t48301\t\"Eddy County, NM\"\t35015\n\"Loving County, TX\"\t48301\t\"Lea County, NM\"\t35025\n\"Loving County, TX\"\t48301\t\"Loving County, TX\"\t48301\n\"Loving County, TX\"\t48301\t\"Reeves County, TX\"\t48389\n\"Loving County, TX\"\t48301\t\"Ward County, TX\"\t48475\n\"Loving County, TX\"\t48301\t\"Winkler County, TX\"\t48495\n\"Lubbock County, TX\"\t48303\t\"Crosby County, TX\"\t48107\n\"Lubbock County, TX\"\t48303\t\"Floyd County, TX\"\t48153\n\"Lubbock County, TX\"\t48303\t\"Garza County, TX\"\t48169\n\"Lubbock County, TX\"\t48303\t\"Hale County, TX\"\t48189\n\"Lubbock County, TX\"\t48303\t\"Hockley County, TX\"\t48219\n\"Lubbock County, TX\"\t48303\t\"Lamb County, TX\"\t48279\n\"Lubbock County, TX\"\t48303\t\"Lubbock County, TX\"\t48303\n\"Lubbock County, TX\"\t48303\t\"Lynn County, TX\"\t48305\n\"Lubbock County, TX\"\t48303\t\"Terry County, TX\"\t48445\n\"Lynn County, TX\"\t48305\t\"Borden County, TX\"\t48033\n\"Lynn County, TX\"\t48305\t\"Crosby County, TX\"\t48107\n\"Lynn County, TX\"\t48305\t\"Dawson County, TX\"\t48115\n\"Lynn County, TX\"\t48305\t\"Garza County, TX\"\t48169\n\"Lynn County, TX\"\t48305\t\"Hockley County, TX\"\t48219\n\"Lynn County, TX\"\t48305\t\"Lubbock County, TX\"\t48303\n\"Lynn County, TX\"\t48305\t\"Lynn County, TX\"\t48305\n\"Lynn County, TX\"\t48305\t\"Terry County, TX\"\t48445\n\"McCulloch County, TX\"\t48307\t\"Brown County, TX\"\t48049\n\"McCulloch County, TX\"\t48307\t\"Coleman County, TX\"\t48083\n\"McCulloch County, TX\"\t48307\t\"Concho County, TX\"\t48095\n\"McCulloch County, TX\"\t48307\t\"McCulloch County, TX\"\t48307\n\"McCulloch County, TX\"\t48307\t\"Mason County, TX\"\t48319\n\"McCulloch County, TX\"\t48307\t\"Menard County, TX\"\t48327\n\"McCulloch County, TX\"\t48307\t\"San Saba County, TX\"\t48411\n\"McLennan County, TX\"\t48309\t\"Bell County, TX\"\t48027\n\"McLennan County, TX\"\t48309\t\"Bosque County, TX\"\t48035\n\"McLennan County, TX\"\t48309\t\"Coryell County, TX\"\t48099\n\"McLennan County, TX\"\t48309\t\"Falls County, TX\"\t48145\n\"McLennan County, TX\"\t48309\t\"Hill County, TX\"\t48217\n\"McLennan County, TX\"\t48309\t\"Limestone County, TX\"\t48293\n\"McLennan County, TX\"\t48309\t\"McLennan County, TX\"\t48309\n\"McMullen County, TX\"\t48311\t\"Atascosa County, TX\"\t48013\n\"McMullen County, TX\"\t48311\t\"Duval County, TX\"\t48131\n\"McMullen County, TX\"\t48311\t\"La Salle County, TX\"\t48283\n\"McMullen County, TX\"\t48311\t\"Live Oak County, TX\"\t48297\n\"McMullen County, TX\"\t48311\t\"McMullen County, TX\"\t48311\n\"McMullen County, TX\"\t48311\t\"Webb County, TX\"\t48479\n\"Madison County, TX\"\t48313\t\"Brazos County, TX\"\t48041\n\"Madison County, TX\"\t48313\t\"Grimes County, TX\"\t48185\n\"Madison County, TX\"\t48313\t\"Houston County, TX\"\t48225\n\"Madison County, TX\"\t48313\t\"Leon County, TX\"\t48289\n\"Madison County, TX\"\t48313\t\"Madison County, TX\"\t48313\n\"Madison County, TX\"\t48313\t\"Robertson County, TX\"\t48395\n\"Madison County, TX\"\t48313\t\"Walker County, TX\"\t48471\n\"Marion County, TX\"\t48315\t\"Caddo Parish, LA\"\t22017\n\"Marion County, TX\"\t48315\t\"Cass County, TX\"\t48067\n\"Marion County, TX\"\t48315\t\"Harrison County, TX\"\t48203\n\"Marion County, TX\"\t48315\t\"Marion County, TX\"\t48315\n\"Marion County, TX\"\t48315\t\"Morris County, TX\"\t48343\n\"Marion County, TX\"\t48315\t\"Upshur County, TX\"\t48459\n\"Martin County, TX\"\t48317\t\"Andrews County, TX\"\t48003\n\"Martin County, TX\"\t48317\t\"Borden County, TX\"\t48033\n\"Martin County, TX\"\t48317\t\"Dawson County, TX\"\t48115\n\"Martin County, TX\"\t48317\t\"Gaines County, TX\"\t48165\n\"Martin County, TX\"\t48317\t\"Glasscock County, TX\"\t48173\n\"Martin County, TX\"\t48317\t\"Howard County, TX\"\t48227\n\"Martin County, TX\"\t48317\t\"Martin County, TX\"\t48317\n\"Martin County, TX\"\t48317\t\"Midland County, TX\"\t48329\n\"Mason County, TX\"\t48319\t\"Gillespie County, TX\"\t48171\n\"Mason County, TX\"\t48319\t\"Kimble County, TX\"\t48267\n\"Mason County, TX\"\t48319\t\"Llano County, TX\"\t48299\n\"Mason County, TX\"\t48319\t\"McCulloch County, TX\"\t48307\n\"Mason County, TX\"\t48319\t\"Mason County, TX\"\t48319\n\"Mason County, TX\"\t48319\t\"Menard County, TX\"\t48327\n\"Mason County, TX\"\t48319\t\"San Saba County, TX\"\t48411\n\"Matagorda County, TX\"\t48321\t\"Brazoria County, TX\"\t48039\n\"Matagorda County, TX\"\t48321\t\"Calhoun County, TX\"\t48057\n\"Matagorda County, TX\"\t48321\t\"Jackson County, TX\"\t48239\n\"Matagorda County, TX\"\t48321\t\"Matagorda County, TX\"\t48321\n\"Matagorda County, TX\"\t48321\t\"Wharton County, TX\"\t48481\n\"Maverick County, TX\"\t48323\t\"Dimmit County, TX\"\t48127\n\"Maverick County, TX\"\t48323\t\"Kinney County, TX\"\t48271\n\"Maverick County, TX\"\t48323\t\"Maverick County, TX\"\t48323\n\"Maverick County, TX\"\t48323\t\"Uvalde County, TX\"\t48463\n\"Maverick County, TX\"\t48323\t\"Webb County, TX\"\t48479\n\"Maverick County, TX\"\t48323\t\"Zavala County, TX\"\t48507\n\"Medina County, TX\"\t48325\t\"Atascosa County, TX\"\t48013\n\"Medina County, TX\"\t48325\t\"Bandera County, TX\"\t48019\n\"Medina County, TX\"\t48325\t\"Bexar County, TX\"\t48029\n\"Medina County, TX\"\t48325\t\"Frio County, TX\"\t48163\n\"Medina County, TX\"\t48325\t\"Medina County, TX\"\t48325\n\"Medina County, TX\"\t48325\t\"Uvalde County, TX\"\t48463\n\"Medina County, TX\"\t48325\t\"Zavala County, TX\"\t48507\n\"Menard County, TX\"\t48327\t\"Concho County, TX\"\t48095\n\"Menard County, TX\"\t48327\t\"Kimble County, TX\"\t48267\n\"Menard County, TX\"\t48327\t\"McCulloch County, TX\"\t48307\n\"Menard County, TX\"\t48327\t\"Mason County, TX\"\t48319\n\"Menard County, TX\"\t48327\t\"Menard County, TX\"\t48327\n\"Menard County, TX\"\t48327\t\"Schleicher County, TX\"\t48413\n\"Menard County, TX\"\t48327\t\"Sutton County, TX\"\t48435\n\"Menard County, TX\"\t48327\t\"Tom Green County, TX\"\t48451\n\"Midland County, TX\"\t48329\t\"Andrews County, TX\"\t48003\n\"Midland County, TX\"\t48329\t\"Ector County, TX\"\t48135\n\"Midland County, TX\"\t48329\t\"Glasscock County, TX\"\t48173\n\"Midland County, TX\"\t48329\t\"Martin County, TX\"\t48317\n\"Midland County, TX\"\t48329\t\"Midland County, TX\"\t48329\n\"Midland County, TX\"\t48329\t\"Reagan County, TX\"\t48383\n\"Midland County, TX\"\t48329\t\"Upton County, TX\"\t48461\n\"Milam County, TX\"\t48331\t\"Bell County, TX\"\t48027\n\"Milam County, TX\"\t48331\t\"Burleson County, TX\"\t48051\n\"Milam County, TX\"\t48331\t\"Falls County, TX\"\t48145\n\"Milam County, TX\"\t48331\t\"Lee County, TX\"\t48287\n\"Milam County, TX\"\t48331\t\"Milam County, TX\"\t48331\n\"Milam County, TX\"\t48331\t\"Robertson County, TX\"\t48395\n\"Milam County, TX\"\t48331\t\"Williamson County, TX\"\t48491\n\"Mills County, TX\"\t48333\t\"Brown County, TX\"\t48049\n\"Mills County, TX\"\t48333\t\"Comanche County, TX\"\t48093\n\"Mills County, TX\"\t48333\t\"Hamilton County, TX\"\t48193\n\"Mills County, TX\"\t48333\t\"Lampasas County, TX\"\t48281\n\"Mills County, TX\"\t48333\t\"Mills County, TX\"\t48333\n\"Mills County, TX\"\t48333\t\"San Saba County, TX\"\t48411\n\"Mitchell County, TX\"\t48335\t\"Borden County, TX\"\t48033\n\"Mitchell County, TX\"\t48335\t\"Coke County, TX\"\t48081\n\"Mitchell County, TX\"\t48335\t\"Fisher County, TX\"\t48151\n\"Mitchell County, TX\"\t48335\t\"Howard County, TX\"\t48227\n\"Mitchell County, TX\"\t48335\t\"Mitchell County, TX\"\t48335\n\"Mitchell County, TX\"\t48335\t\"Nolan County, TX\"\t48353\n\"Mitchell County, TX\"\t48335\t\"Scurry County, TX\"\t48415\n\"Mitchell County, TX\"\t48335\t\"Sterling County, TX\"\t48431\n\"Montague County, TX\"\t48337\t\"Jefferson County, OK\"\t40067\n\"Montague County, TX\"\t48337\t\"Love County, OK\"\t40085\n\"Montague County, TX\"\t48337\t\"Clay County, TX\"\t48077\n\"Montague County, TX\"\t48337\t\"Cooke County, TX\"\t48097\n\"Montague County, TX\"\t48337\t\"Jack County, TX\"\t48237\n\"Montague County, TX\"\t48337\t\"Montague County, TX\"\t48337\n\"Montague County, TX\"\t48337\t\"Wise County, TX\"\t48497\n\"Montgomery County, TX\"\t48339\t\"Grimes County, TX\"\t48185\n\"Montgomery County, TX\"\t48339\t\"Harris County, TX\"\t48201\n\"Montgomery County, TX\"\t48339\t\"Liberty County, TX\"\t48291\n\"Montgomery County, TX\"\t48339\t\"Montgomery County, TX\"\t48339\n\"Montgomery County, TX\"\t48339\t\"San Jacinto County, TX\"\t48407\n\"Montgomery County, TX\"\t48339\t\"Walker County, TX\"\t48471\n\"Montgomery County, TX\"\t48339\t\"Waller County, TX\"\t48473\n\"Moore County, TX\"\t48341\t\"Carson County, TX\"\t48065\n\"Moore County, TX\"\t48341\t\"Dallam County, TX\"\t48111\n\"Moore County, TX\"\t48341\t\"Hansford County, TX\"\t48195\n\"Moore County, TX\"\t48341\t\"Hartley County, TX\"\t48205\n\"Moore County, TX\"\t48341\t\"Hutchinson County, TX\"\t48233\n\"Moore County, TX\"\t48341\t\"Moore County, TX\"\t48341\n\"Moore County, TX\"\t48341\t\"Oldham County, TX\"\t48359\n\"Moore County, TX\"\t48341\t\"Potter County, TX\"\t48375\n\"Moore County, TX\"\t48341\t\"Sherman County, TX\"\t48421\n\"Morris County, TX\"\t48343\t\"Bowie County, TX\"\t48037\n\"Morris County, TX\"\t48343\t\"Camp County, TX\"\t48063\n\"Morris County, TX\"\t48343\t\"Cass County, TX\"\t48067\n\"Morris County, TX\"\t48343\t\"Marion County, TX\"\t48315\n\"Morris County, TX\"\t48343\t\"Morris County, TX\"\t48343\n\"Morris County, TX\"\t48343\t\"Red River County, TX\"\t48387\n\"Morris County, TX\"\t48343\t\"Titus County, TX\"\t48449\n\"Morris County, TX\"\t48343\t\"Upshur County, TX\"\t48459\n\"Motley County, TX\"\t48345\t\"Briscoe County, TX\"\t48045\n\"Motley County, TX\"\t48345\t\"Cottle County, TX\"\t48101\n\"Motley County, TX\"\t48345\t\"Crosby County, TX\"\t48107\n\"Motley County, TX\"\t48345\t\"Dickens County, TX\"\t48125\n\"Motley County, TX\"\t48345\t\"Floyd County, TX\"\t48153\n\"Motley County, TX\"\t48345\t\"Hall County, TX\"\t48191\n\"Motley County, TX\"\t48345\t\"King County, TX\"\t48269\n\"Motley County, TX\"\t48345\t\"Motley County, TX\"\t48345\n\"Nacogdoches County, TX\"\t48347\t\"Angelina County, TX\"\t48005\n\"Nacogdoches County, TX\"\t48347\t\"Cherokee County, TX\"\t48073\n\"Nacogdoches County, TX\"\t48347\t\"Nacogdoches County, TX\"\t48347\n\"Nacogdoches County, TX\"\t48347\t\"Rusk County, TX\"\t48401\n\"Nacogdoches County, TX\"\t48347\t\"San Augustine County, TX\"\t48405\n\"Nacogdoches County, TX\"\t48347\t\"Shelby County, TX\"\t48419\n\"Navarro County, TX\"\t48349\t\"Ellis County, TX\"\t48139\n\"Navarro County, TX\"\t48349\t\"Freestone County, TX\"\t48161\n\"Navarro County, TX\"\t48349\t\"Henderson County, TX\"\t48213\n\"Navarro County, TX\"\t48349\t\"Hill County, TX\"\t48217\n\"Navarro County, TX\"\t48349\t\"Limestone County, TX\"\t48293\n\"Navarro County, TX\"\t48349\t\"Navarro County, TX\"\t48349\n\"Newton County, TX\"\t48351\t\"Beauregard Parish, LA\"\t22011\n\"Newton County, TX\"\t48351\t\"Calcasieu Parish, LA\"\t22019\n\"Newton County, TX\"\t48351\t\"Sabine Parish, LA\"\t22085\n\"Newton County, TX\"\t48351\t\"Vernon Parish, LA\"\t22115\n\"Newton County, TX\"\t48351\t\"Jasper County, TX\"\t48241\n\"Newton County, TX\"\t48351\t\"Newton County, TX\"\t48351\n\"Newton County, TX\"\t48351\t\"Orange County, TX\"\t48361\n\"Newton County, TX\"\t48351\t\"Sabine County, TX\"\t48403\n\"Nolan County, TX\"\t48353\t\"Coke County, TX\"\t48081\n\"Nolan County, TX\"\t48353\t\"Fisher County, TX\"\t48151\n\"Nolan County, TX\"\t48353\t\"Jones County, TX\"\t48253\n\"Nolan County, TX\"\t48353\t\"Mitchell County, TX\"\t48335\n\"Nolan County, TX\"\t48353\t\"Nolan County, TX\"\t48353\n\"Nolan County, TX\"\t48353\t\"Runnels County, TX\"\t48399\n\"Nolan County, TX\"\t48353\t\"Scurry County, TX\"\t48415\n\"Nolan County, TX\"\t48353\t\"Taylor County, TX\"\t48441\n\"Nueces County, TX\"\t48355\t\"Aransas County, TX\"\t48007\n\"Nueces County, TX\"\t48355\t\"Jim Wells County, TX\"\t48249\n\"Nueces County, TX\"\t48355\t\"Kleberg County, TX\"\t48273\n\"Nueces County, TX\"\t48355\t\"Nueces County, TX\"\t48355\n\"Nueces County, TX\"\t48355\t\"San Patricio County, TX\"\t48409\n\"Ochiltree County, TX\"\t48357\t\"Beaver County, OK\"\t40007\n\"Ochiltree County, TX\"\t48357\t\"Texas County, OK\"\t40139\n\"Ochiltree County, TX\"\t48357\t\"Hansford County, TX\"\t48195\n\"Ochiltree County, TX\"\t48357\t\"Lipscomb County, TX\"\t48295\n\"Ochiltree County, TX\"\t48357\t\"Ochiltree County, TX\"\t48357\n\"Ochiltree County, TX\"\t48357\t\"Roberts County, TX\"\t48393\n\"Oldham County, 
